vi "Filter Control.vi"(8 "control_current_filter_index":dbl, 10 "control_laser_source":string, 11 "control_request":string) -> (3 "indicator_filter_status":bool)   [LabVIEW 2020]
uses:
  <vilib>/Utility/file.llb/Read Delimited Spreadsheet (string).vi
panel:
  out "error out 3":errorcluster
  out "error out 2":errorcluster
  out "error out":errorcluster
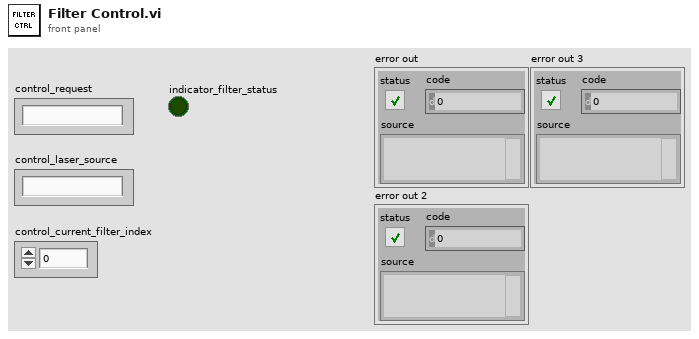
[diagram p1: front panel]
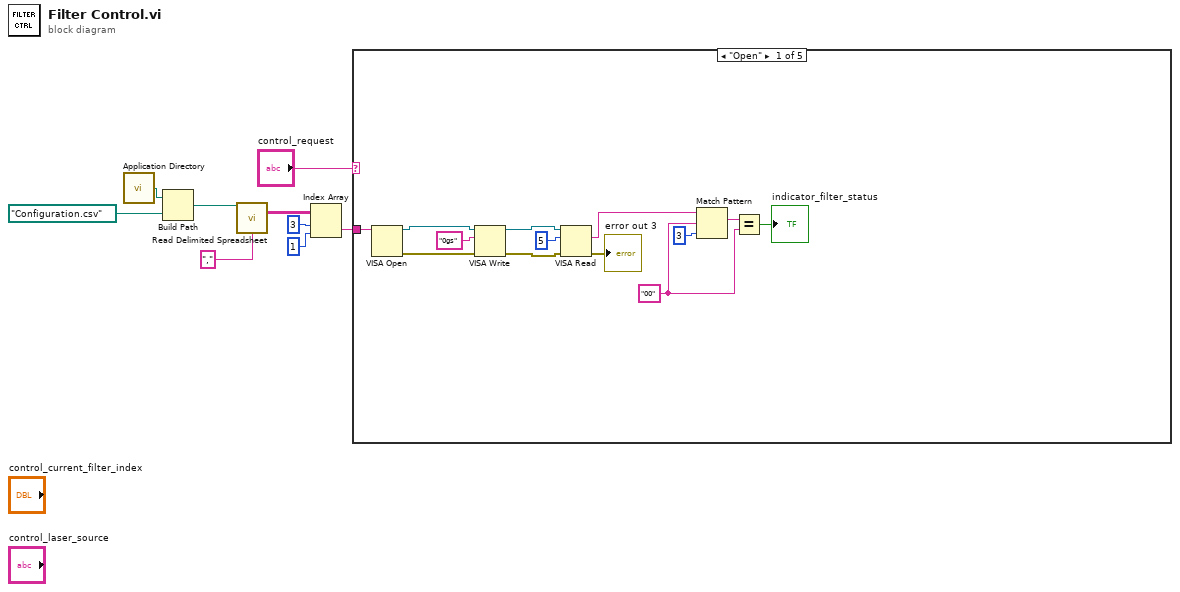
[diagram p0: block diagram]
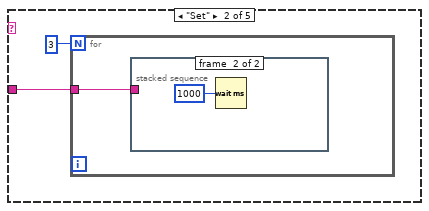
[diagram p2: hidden frame]
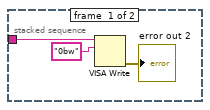
[diagram p3: hidden frame]
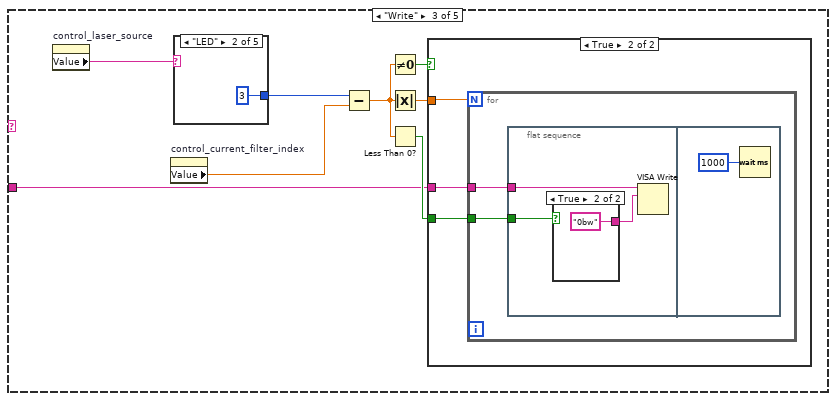
[diagram p4: hidden frame]
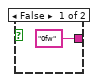
[diagram p6: hidden frame]
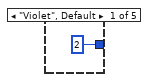
[diagram p7: hidden frame]
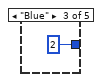
[diagram p8: hidden frame]
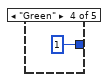
[diagram p9: hidden frame]
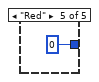
[diagram p10: hidden frame]
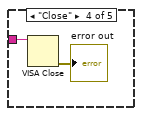
[diagram p11: hidden frame]
diagram:
  n1 = call <vilib>:"Application Directory.vi"() -> ("Application Directory"=w5:path)
  n2 = Build Path(base path=w5, name or relative path=path "Configuration.csv" ("file path (dialog if empty)")) -> (appended path=w4:path)
  n3 = call-poly <vilib>:"Read Delimited Spreadsheet.vi"("file path (dialog if empty)"=w4, "delimiter (\\t)"="," ("delimiter (\\t)")) -> ("all rows"=w2:string[][])  [unwired: 8 in, 5 out]
  n4 = Index Array(array=w2, index (row)=3, index (col)=1 ("disabled index (col)")) -> (element=w1:string)
  n5 = case shown="\"Open\"" "control_request" {
    tunnel: w1 -> [w22 w24 w30 w55 _]
    frame "Open" {
      w14 = "00" ("regular expression")
      n6 = VISA Open(VISA resource name=w22) -> (VISA resource name=w20:refnum<visa-resource-name>, error out=w21:errorcluster)  [unwired: 4 in]
      n7 = VISA Write(VISA resource name=w20, write buffer="0gs", error in (no error)=w21) -> (VISA resource name out=w15:refnum<visa-resource-name>, error out=w19:errorcluster)  [unwired: 1 out]
      n8 = VISA Read(VISA resource name=w15, byte count=u32 5, error in (no error)=w19) -> (read buffer=w16:string, error out=→"error out 3":errorcluster)  [unwired: 2 out]
      n9 = Match Pattern(string=w16, regular expression=w14, offset (0)=3) -> (match substring=w17:string)  [unwired: 3 out]
      n10 = Equal?(x=w17, y=w14) -> (x = y?=→"indicator_filter_status":bool)
    }
    frame "Set" {
      n11 = for {
        N: 3 -> [_]
        tunnel: w24 -> [w25]
        n12 = stacked-sequence {
          tunnel: w25 -> [w27 _]
          frame #0 {
            n13 = VISA Write(VISA resource name=w27, write buffer="0bw") -> (error out=→"error out 2":errorcluster)  [unwired: 1 in, 2 out]
          }
          frame #1 {
            n14 = Wait (ms)(milliseconds to wait=u32 1000) -> ()  [unwired: 1 out]
          }
        }
      }
    }
    frame "Write" {
      n15 = property on="control_laser_source" class="Str"() -> ("Value"=w31:string)  [unwired: 2 in, 2 out]
      n16 = property on="control_current_filter_index" class="DigNum (strict)"() -> ("Value"=w36:dbl)  [unwired: 2 in, 2 out]
      n17 = case shown="\"LED\"" w31 {
        tunnel: [2 3 2 1 0] -> w37
        frame "Violet", Default {
        }
        frame "LED" {
        }
        frame "Blue" {
        }
        frame "Green" {
        }
        frame "Red" {
        }
      }
      n18 = Subtract(x=w37, y=w36) -> (x-y=w33:dbl)
      n19 = Not Equal To 0?(x=w33) -> (x != 0?=w35:bool)
      n20 = Absolute Value(x=w33) -> (abs(x)=w34:dbl)
      n21 = Less Than 0?(x=w33) -> (x < 0?=w32:bool)
      n22 = case shown="True" w35 {
        tunnel: w34 -> [_ w40]
        tunnel: w32 -> [_ w39]
        tunnel: w30 -> [_ w38]
        frame False {
        }
        frame True {
          n23 = for {
            N: w40 -> [_]
            tunnel: w39 -> [w42]
            tunnel: w38 -> [w41]
            n24 = flat-sequence {
              tunnel: w42 -> [w44]
              tunnel: w41 -> [w43]
              frame #0 {
                n25 = case shown="True" w44 {
                  tunnel: ["0fw" ("write buffer") "0bw" ("write buffer")] -> w45
                  frame False {
                  }
                  frame True {
                  }
                }
                n26 = VISA Write(VISA resource name=w43, write buffer=w45) -> ()  [unwired: 1 in, 3 out]
              }
              frame #1 {
                n27 = Wait (ms)(milliseconds to wait=u32 1000) -> ()  [unwired: 1 out]
              }
            }
          }
        }
      }
    }
    frame "Close" {
      n28 = VISA Close(VISA resource name=w55) -> (error out=→"error out":errorcluster)  [unwired: 1 in]
    }
    frame "Default", Default {
    }
  }
